vi "FTW-CodeGen-FindTerm-Ref.vi"(5 "Terms":T1(array[cluster]), 7 "Terminal ID":string) -> (6 "Terminal Ref":refnum<vi>, 8 "Found?":bool)   [LabVIEW 2015]
panel:
  # "Inputs"
  # "Outputs"
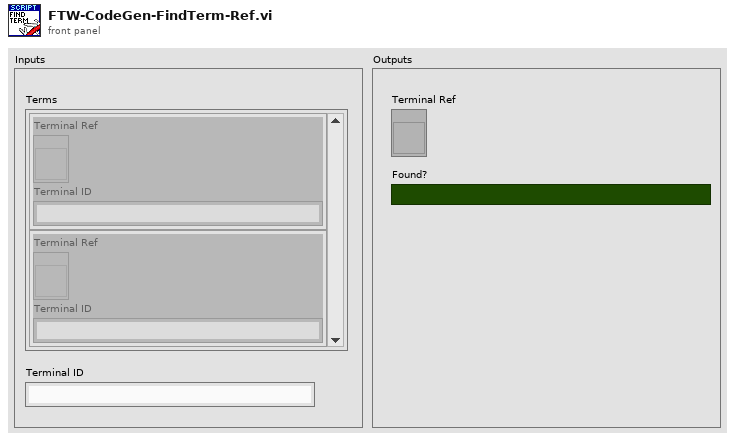
[diagram p1: front panel]
types:
  T1 = cluster{"Terminal Ref":refnum<vi>, "Terminal ID":string}[]
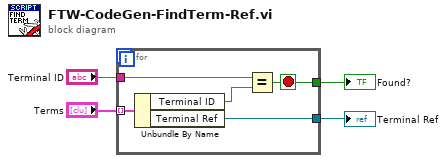
[diagram p0: block diagram]
diagram:
  n1 = for {
    tunnel: [w9] -> w2
    tunnel: [w8] -> w4
    tunnel: "Terms" -> [w7] mode=indexing
    tunnel: "Terminal ID" -> [w5]
    stop <- w8 stop-if-true
    n2 = Unbundle By Name(w7) -> ("Terminal ID"=w6:string, "Terminal Ref"=w9:refnum<vi>)
    n3 = Equal?(x=w5, y=w6) -> (x = y?=w8:bool)
  }
  "Terminal Ref" <- w2
  "Found?" <- w4
